vi "vna query opc.vi"(8 "error in (no error)":errorcluster, 11 "VISA resource name":refnum<visa-resource-name>) -> (0 "error out":errorcluster, 3 "VISA resource name 2":refnum<visa-resource-name>)   [LabVIEW 2013]
panel:
  out "error tmp":errorcluster
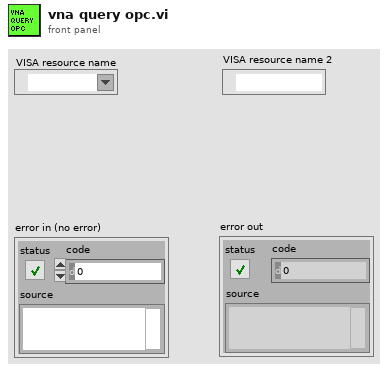
[diagram p1: front panel]
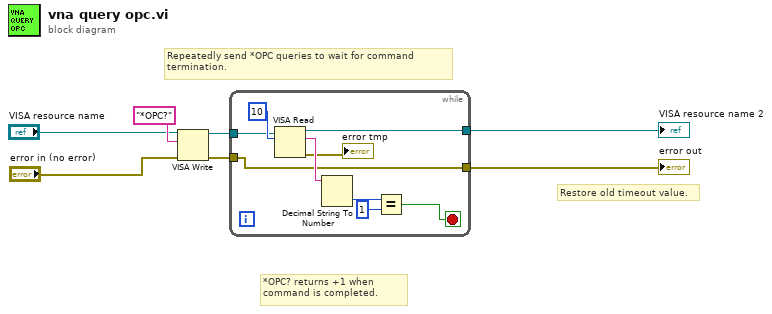
[diagram p0: block diagram]
diagram:
  # "Restore old timeout value."
  # "*OPC? returns +1 when command is completed."
  # "Repeatedly send *OPC queries to wait for command termination."
  n1 = VISA Write(VISA resource name="VISA resource name", write buffer="*OPC?", error in (no error)="error in (no error)") -> (VISA resource name out=w3:refnum<visa-resource-name>, error out=w4:errorcluster)  [unwired: 1 out]
  n2 = while {
    tunnel: [w11] -> w1
    tunnel: w4 -> [w8]
    tunnel: w3 -> [w9]
    tunnel: [w8] -> w2
    stop <- w12 stop-if-true
    n3 = VISA Read(VISA resource name=w9, byte count=u32 10) -> (VISA resource name out=w11:refnum<visa-resource-name>, read buffer=w15:string, error out=→"error tmp":errorcluster)  [unwired: 1 in, 1 out]
    n4 = Decimal String To Number(string=w15) -> (number=w14:i32)  [unwired: 2 in, 1 out]
    n5 = Equal?(x=w14, y=1) -> (x = y?=w12:bool)
  }
  "VISA resource name 2" <- w1
  "error out" <- w2
